vi "evo irimager get thermal image.vi"(10 "h":i32, 11 "w":i32) -> (0 "data out":u16[](array[numeric]), 2 "h out":i32, 3 "w out":i32, 5 "function return":i32)   [LabVIEW 2025, in "libirimager_direct_binding.lvlib"]
doc: "DIRECT_API int evo_irimager_get_thermal_image(int* w, int* h, unsigned short* data);"
uses:
  libirimager_direct_binding.lvlib
  libirimager.dll
panel:
  out "flagState":T1(ring)
  out "tempBox":sgl
  out "tempFlag":sgl
  out "tempChip":sgl
  out "timestampMedia":i64
  out "timestamp":i64
  out "counterHW":u32
  out "counter":u32
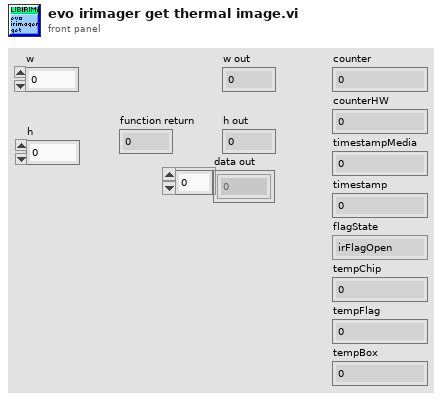
[diagram p1: front panel]
types:
  T1 = enum32{"irFlagOpen", "irFlagClose", "irFlagOpening", "irFlagClosing", "irFlagError"}
  T2 = cluster{"counter":u32, "counterHW":u32, "timestamp":i64, "timestampMedia":i64, "flagState":enum32{"irFlagOpen", "irFlagClose", "irFlagOpening", "irFlagClosing", "irFlagError"}, "tempChip":sgl, "tempFlag":sgl, "tempBox":sgl}
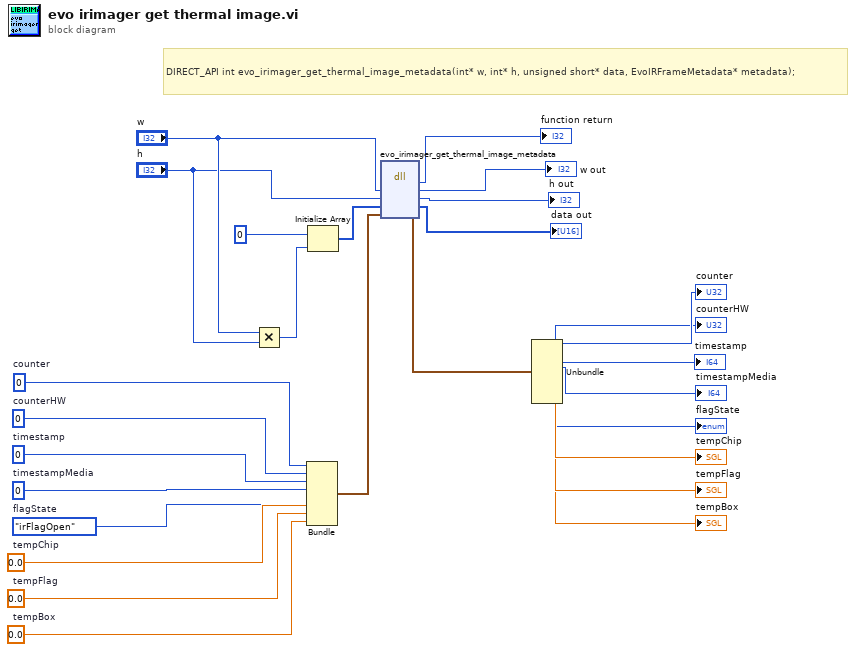
[diagram p0: block diagram]
diagram:
  w2 = T1."irFlagOpen"  # flagState
  w12 = sgl 0.0  # tempBox
  w13 = sgl 0.0  # tempFlag
  w14 = sgl 0.0  # tempChip
  w15 = i64 0  # timestampMedia
  w16 = i64 0  # timestamp
  w11 = u32 0  # counterHW
  w10 = u32 0  # counter
  # "DIRECT_API int evo_irimager_get_thermal_image_metadata(int* w, int* h, unsigned short* data, EvoIRFrameMetadata* metadata);"
  n1 = Multiply(x="w", y="h") -> (x*y=w23:i32)
  n2 = Bundle("counter"=w10, "counterHW"=w11, "timestamp"=w16, "timestampMedia"=w15, "flagState"=w2, "tempChip"=w14, "tempFlag"=w13, "tempBox"=w12) -> (w3:T2)  [unwired: 1 in]
  n3 = Initialize Array(0, w23) -> (w19:i32[])
  n4 = dll-call lib="C:/Users/mayhe/OneDrive/Documents/GitHub/In-situ-monitoring-of-powder-bed-fusion-additive-manufacturing/system_development/Adamant/v0.2/software_development/thermal-camera/VI/labview/libirimager.dll" fn="evo_irimager_get_thermal_image_metadata"("w"="w", "h"="h", "data"=w19, "metadata"=w3) -> ("Rückgabetyp"=→"function return":i32, "w"=→"w out":i32, "h"=→"h out":i32, "data"=→"data out":u16[], "metadata"=w17:T2)  [unwired: 3 in, 2 out]
  n5 = Unbundle(w17) -> ("counter"=→"counter":u32, "counterHW"=→"counterHW" →"timestamp":u32, "timestampMedia"=→"timestampMedia":i64, "flagState"=→"flagState":T1, "tempChip"=→"tempChip":sgl, "tempFlag"=→"tempFlag":sgl, "tempBox"=→"tempBox":sgl)  [unwired: 1 out]
